vi "Move_two_axis.vi"(2 "Pulse Number 2":i32=100 min=1 max=500000, 3 "Pulse Number 1":i32=100 min=1 max=500000, 4 "Residence time":i32=100 min=1 max=500000, 5 "Port Number":i8=7 min=0) -> (0 "OK Done":bool=TRUE, 1 "String Received":string="OK\r\n")   [LabVIEW 2013]
panel:
  out "Received String2":string="R\r\n"
  out "Command String":string="A:W+P1000+P1000"
  # "Port Number 0=COM1"
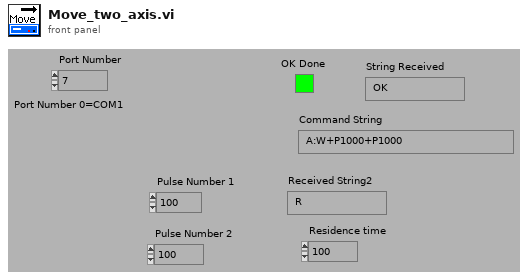
[diagram p1: front panel]
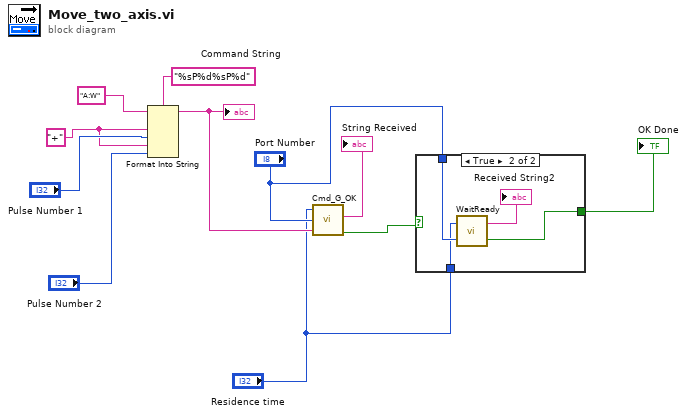
[diagram p0: block diagram]
diagram:
  w2 = "+"
  n1 = Format Into String(format string="%sP%d%sP%d", initial string="A:W", w2, "Pulse Number 1", w2, "Pulse Number 2") -> (resulting string=w9:string)  [unwired: 1 in, 1 out]
  "Command String" <- w9
  n2 = call "Cmd_G_OK.vi"("Residence time"="Residence time", "PortNumber"="Port Number", "Command String"=w9) -> ("Received String2"=→"String Received":string, "OK Done"=w6:bool)  [unwired: 2 out]
  n3 = case shown="True" w6 {
    selector: w6 -> [w12 _]
    tunnel: "Port Number" -> [_ w16]
    tunnel: [w12 w14] -> w5
    tunnel: "Residence time" -> [_ w13]
    frame False {
    }
    frame True {
      n4 = call "WaitReady.vi"("PortNumber"=w16, "Residence time in ms"=w13) -> ("OK Done"=w14:bool, "String Received"=→"Received String2":string)
    }
  }
  "OK Done" <- w5
